vi "ReversedEngineering UpdateAttributes.vi"(1 "ClassPath/LvClassRef":variant, 2 "NewAttributes":string="Sträng:STRING\nMittCluster:CLUSTER", 3 "ClassInfo":cluster{"ClassNamn":string, "ClassPath":path}[](array[cluster]), 5 "error in (no error)":errorcluster, 6 "Don't Prompt (False)":bool, 7 "Attributes":T1[](array[typedef]), 8 "Stereotype":string) -> (18 "Cancel":bool=TRUE, 19 "error out":errorcluster)   [LabVIEW 2012] (continued)
"Recessed Up Triangle"=3618, "Reciprocal"=1059, "Reciprocal Of Pi"=2017, "Reciprocal Of e"=2021, "Rectangular Stop Button"=3128, "Refnum to Path"=1424, "Refnum to Session"=2306, "Register Event Callback"=2078, "Register For Events"=2065, "Register Session"=2319, "Release Notifier"=9102, "Release Queue"=9109, "Replace Array Subset"=3910, "Replace Substring"=3913, "Request Deallocation"=1610, "ResetSys"=1976, "Reshape Array"=2055, "Reverse 1D Array"=1900, "Reverse String"=1537, "Right Arrow"=3825, "Right Bow Valve"=21765, "Right Bow Valve 1"=3705, "Right Bow Valve 2"=3805, "Right Down Elbow"=3817, "Right Down Elbow 1"=3717, "Right Pump"=3719, "Right Pump 1"=3819, "Right Rect Valve"=3804, "Right Rect Valve 1"=3704, "Right Rect Valve 2"=21764, "Right Tee"=3715, "Right Tee 1"=3815, "Right Up Elbow"=3814, "Right Up Elbow 1"=3714, "Ring Constant"=2008, "Rocker"=21002, "Rotary Feeder"=3830, "Rotate"=1082, "Rotate 1D Array"=1906, "Rotate Left With Carry"=1606, "Rotate Right With Carry"=1607, "Rotate String"=1536, "Round Button"=3100, "Round LED"=21012, "Round LED 1"=3120, "Round Light"=3104, "Round Push Button"=3112, "Round Push Button 2"=3118, "Round Radio Button"=3106, "Round Stop Button"=3127, "Round To +Infinity"=1076, "Round To -Infinity"=1075, "Round To Nearest"=1055, "Rydberg Constant (/m)"=2031, "Scale By Power Of 2"=1074, "Scan From File"=2082, "Scan From String"=2080, "Scan String For Tokens"=8101, "Scan Value"=1534, "Search 1D Array"=1901, "Search and Replace String"=3914, "Search/Split String"=1538, "Secant"=1203, "Seconds To Date/Time"=1309, "Seek"=1409, "Select"=1516, "Send"=1977, "Send Notification"=9104, "SendCmds"=1978, "SendDataBytes"=1979, "SendIFC"=1980, "SendLLO"=1982, "SendList"=1981, "SendSetup"=1983, "Session to Refnum"=2307, "Set Menu Item Info"=9006, "Set Occurrence"=1702, "Set Variant Attribute"=8204, "Set Waveform Attribute"=8207, "SetRWLS"=1984, "SetTimeOut"=1985, "Sign"=1049, "Simple Horizontal Slide"=3003, "Simple Numeric"=2900, "Simple Numeric 1"=3029, "Simple String"=2115, "Simple Vertical Slide"=3002, "Simulation Loop"=2099, "Sinc"=1227, "Sine"=1200, "Sine & Cosine"=1220, "Single Selection Listbox"=21200, "Size Handle"=1603, "Slide Switch"=21011, "Sort 1D Array"=1120, "Speed Of Light In Vacuum (m/sec)"=2028, "Split 1D Array"=1908, "Split Button"=21020, "Split Number"=1170, "Split Signals"=2351, "Spreadsheet String To Array"=1539, "Square Button"=3101, "Square LED"=3121, "Square LED 1"=21013, "Square Light"=3105, "Square Push Button"=3113, "Square Push Button 2"=3119, "Square Radio Button"=3107, "Square Root"=1060, "Stacked Sequence Structure"=2000, "Standard ListBox"=3202, "State Diagram"=2051, "Static VI Reference"=2084, "Stop"=1350, "Stop Button"=21230, "String Constant"=2007, "String Control"=3200, "String Control 1"=21701, "String Indicator"=3201, "String Indicator 1"=21702, "String Length"=1502, "String Subset"=1503, "String To Byte Array"=1608, "String To IP"=1711, "String To Path"=1078, "String to Tag"=1830, "Strip Path"=1420, "SubPanel"=21810, "SubPanel (Classic)"=21811, "Subtract"=1051, "Swap Bytes"=1162, "Swap Vector Element"=1912, "Swap Words"=1163, "TCP Close Connection"=1713, "TCP Create Listener"=1717, "TCP Flattened Read"=1718, "TCP Flattened Write"=1719, "TCP Flex Read"=1720, "TCP Flex Write"=1721, "TCP Network Connection Refnum"=3407, "TCP Open Connection"=1715, "TCP Read"=1716, "TCP Wait On Listener"=1712, "TCP Write"=1714, "Tab Constant"=2012, "Tab Control"=3332, "Tab Control 1"=3330, "Table"=3301, "Table 1"=21202, "Table 2"=21212, "Tag Attribute Ring"=2063, "Tag Constant"=2089, "Tag Control"=21742, "Tag Control 1"=3302, "Tag Indicator"=21743, "Tag Indicator 1"=3303, "Tag to String"=1831, "Tangent"=1202, "Tank"=3020, "Tank 1"=21006, "Temporary Directory"=1435, "TestSRQ"=1986, "TestSys"=1987, "Text & Pict Ring"=21603, "Text & Pict Ring 1"=3016, "Text Button"=21015, "Text Ring"=21601, "Text Ring 1"=3014, "Thermometer"=21007, "Thermometer 1"=3021, "Thick Chiseled Line"=3630, "Thick Line"=3629, "Thick Line with Arrow"=3631, "Thick Lowered Box"=3635, "Thin Chiseled Line"=3627, "Thin Line"=3626, "Thin Line with Arrow"=3628, "Threshold 1D Array"=1909, "Tick Count (ms)"=1300, "Time Stamp Constant"=2068, "Time Stamp Control"=5555, "Time Stamp Control 1"=21913, "Time Stamp Indicator"=5556, "Time Stamp Indicator 1"=21914, "Timed Loop"=5570, "To Byte Integer"=1140, "To Double Precision Complex"=1152, "To Double Precision Float"=1147, "To Extended Precision Complex"=1154, "To Extended Precision Float"=1149, "To Long Integer"=1142, "To Lower Case"=1189, "To More Generic Class"=8017, "To More Specific Class"=8016, "To OLE Variant"=8002, "To Quad Integer"=1155, "To Single Precision Complex"=1151, "To Single Precision Float"=1146, "To Time Stamp"=5560, "To Unsigned Byte Integer"=1143, "To Unsigned Long Integer"=1145, "To Unsigned Quad Integer"=1156, "To Unsigned Word Integer"=1144, "To Upper Case"=1188, "To Variant"=8201, "To Word Integer"=1141, "Traditional DAQ Channel"=21733, "Traditional DAQ Channel 1"=3320, "Traditional DAQ Channel Constant"=2085, "Transpose 2D Array"=1902, "Tree"=21793, "Trigger"=1988, "TriggerList"=1989, "Two Button Dialog"=1341, "Type Cast"=1166, "Type and Creator"=1434, "UDP Close"=1726, "UDP Multicast Open"=1727, "UDP Network Connection Refnum"=3418, "UDP Open"=1723, "UDP Read"=1724, "UDP Write"=1725, "Unbundle"=2048, "Unbundle By Name"=2058, "Unflatten From String"=1161, "Unflatten From XML"=8401, "Uniform Dbl Waveform"=3312, "Uniform Int16 Waveform"=3313, "Unregister For Events"=2076, "Unregister Session"=2320, "Up Arrow"=3823, "Up Bow Valve"=3703, "Up Bow Valve 1"=21763, "Up Bow Valve 2"=3803, "Up Rect Valve"=21762, "Up Rect Valve 1"=3702, "Up Rect Valve 2"=3802, "Up Tee"=3812, "Up Tee 1"=3712, "User Item"=3506, "VI Library"=1425, "VI Refnum"=3422, "VISA Assert Interrupt Signal"=2309, "VISA Assert Trigger"=1929, "VISA Assert Utility Signal"=2310, "VISA Clear"=1927, "VISA Close"=1922, "VISA Disable Event"=1940, "VISA Discard Events"=1941, "VISA Enable Event"=1942, "VISA Find Resource"=1923, "VISA Flush I/O Buffer"=2302, "VISA GPIB Command"=2315, "VISA GPIB Control ATN"=2316, "VISA GPIB Control REN"=2304, "VISA GPIB Pass Control"=2317, "VISA GPIB Send IFC"=2318, "VISA In 16"=1930, "VISA In 32"=1944, "VISA In 8"=1936, "VISA Lock"=1993, "VISA Map Address"=1932, "VISA Map Trigger"=2311, "VISA Memory Allocation"=1997, "VISA Memory Free"=1998, "VISA Move"=2303, "VISA Move In 16"=1948, "VISA Move In 32"=1991, "VISA Move In 8"=1946, "VISA Move Out 16"=1949, "VISA Move Out 32"=1992, "VISA Move Out 8"=1947, "VISA Open"=2308, "VISA Out 16"=1931, "VISA Out 32"=1945, "VISA Out 8"=1937, "VISA Peek 16"=1934, "VISA Peek 32"=1995, "VISA Peek 8"=1938, "VISA Poke 16"=1935, "VISA Poke 32"=1996, "VISA Poke 8"=1939, "VISA Read"=1925, "VISA Read STB"=1928, "VISA Read To File"=2313, "VISA Refnum to Session"=2300, "VISA Resource Name"=21737, "VISA Resource Name Constant"=3421, "VISA Set I/O Buffer Size"=2301, "VISA Status Description"=1924, "VISA USB Control In"=2086, "VISA USB Control Out"=2087, "VISA Unlock"=1994, "VISA Unmap Address"=1933, "VISA Unmap Trigger"=2312, "VISA VXI Cmd or Query"=2305, "VISA Wait on Event"=1943, "VISA Write"=1926, "VISA Write From File"=2314, "VISA resource name"=3409, "Variant"=3310, "Variant To Data"=8003, "Variant To Flattened String"=8203, "Vert Line"=3822, "Vert Pipe"=3716, "Vert Pipe 1"=3816, "Vert Rocker"=21740, "Vertical Fill Slide"=21014, "Vertical Fill Slide 1"=3009, "Vertical Graduated Bar"=21107, "Vertical Pointer Slide"=21017, "Vertical Pointer Slide 1"=3007, "Vertical Progress Bar"=21104, "Vertical Slide"=3004, "Vertical Slide Switch"=21741, "Vertical Slide Switch 1"=3115, "Vertical Smooth Box"=3634, "Vertical Switch"=3109, "Vertical Toggle Switch"=21005, "Vertical Toggle Switch 1"=3111, "Volume Info"=1414, "Wait (ms)"=1302, "Wait For Activity"=1722, "Wait For Front Panel Activity"=1328, "Wait Until Next ms Multiple"=1327, "Wait for GPIB RQS"=1952, "Wait on Notification"=9105, "Wait on Notification from Multiple"=9106, "Wait on Occurrence"=1701, "WaitSRQ"=1990, "Waveform Chart"=3501, "Waveform Chart 1"=21717, "Waveform Chart 2"=21010, "Waveform Graph"=21703, "Waveform Graph 1"=3504, "While Loop"=2003, "While Loop 1"=2352, "White Space?"=1125, "Write Device"=1431, "Write File"=1408, "XY Graph"=3500, "XY Graph 1"=21716, "Xmath Script"=9022]
            n131 = Unbundle By Name(w370) -> ("BaseClassType"=w360:i16[], "OrgCtrl"=w365:refnum<vi>)
            n132 = property class="VI"(reference=w365, error in=w364) -> ("Callees' Names"=w362:string[])  [unwired: 2 out]
            n133 = Array Size(array=w362) -> (size(s)=w361:i32)
            n134 = while {
              tunnel: [w397] -> w374
              tunnel: w362 -> [w382] mode=indexing
              tunnel: [w396] -> w363
              tunnel: w361 -> [w393]
              tunnel: w360 -> [w385]
              i -> [w394]
              stop <- w392 stop-if-true
              n135 = call <resource>:"CommonVIs_UmlOpenVIRef.vi"("ViPath/ViName"=w382) -> ("error out"=w381:errorcluster, "vi reference"=w380:refnum<vi>)  [unwired: 3 in, 6 out]
              n136 = Increment(x=w394) -> (x+1=w395:i32)
              n137 = Greater Or Equal?(x=w395, y=w393) -> (x >= y?=w383:bool)
              n138 = property class="VI"(reference=w380, error in=w381) -> (reference out=w399:refnum<vi>, error out=w398:errorcluster, "VI Path"=w397:path, "Front Panel"=w391:refnum<vi>)
              n139 = property class="Pnl"(reference=w391) -> ("Controls[]"=w390:refnum<vi>[])  [unwired: 1 in, 2 out]
              n140 = Index Array(array=w390) -> (element=w389:refnum<vi>)  [unwired: 1 in]
              n141 = property class="Ctl"(reference=w389) -> ("Type Descriptor"=w388:i16[], "Label.Text"=w387:string)  [unwired: 1 in, 2 out]
              n142 = Close Reference(reference=w399, error in (no error)=w398) -> (error out=w396:errorcluster)
              n143 = call <resource>:"ReversedEngineering TypeDescNonNameDepentent.vi"("Type DescriptorNameDependent"=w388, "LabelText"=w387) -> ("Type DescriptorNonNameDependent"=w386:i16[])  [unwired: 17 out]
              n144 = Equal?(x=w385, y=w386) -> (x = y?=w384:bool)
              n145 = Or(x=w383, y=w384) -> (x .or. y?=w392:bool)
            }
            n146 = Unbundle By Name(w370) -> ("NewCluster"=w375:refnum<vi>)
            n147 = New VI Object(vi object class=w376, owner refnum=w375, style=w377, position/next to=cluster{"Horizontal":i16, "Vertical":i16} {"Horizontal"=0, "Vertical"=0}, 6:w374, 8:w363) -> (object refnum=w378:refnum<vi>, 0:w372:errorcluster)  [unwired: 2 out]
            n148 = property class="Clust"(reference=w378, error in=w372, "Label.Visible"=TRUE) -> (reference out=w368:refnum<vi>, error out=w366:errorcluster)
            n149 = Build Array(w368) -> (w367:refnum<vi>[])
            n150 = Bundle By Name(cluster=w370, "AddedCtrls"=w367) -> (w369:T4)
          }
          frame "GetOrgCtrlMembers" {
            (unwired) CommonVIs_AttributeDataType."UINT8" ("AttributeDataType")
            (unwired) CommonVIs_AttributeDataType."UINT8" ("type")
            n151 = Unbundle By Name(w408) -> ("OrgCluster"=w412:refnum<vi>)
            n152 = property class="Clust"(reference=w412, error in=w409) -> (error out=w410:errorcluster, "Controls[]"=w406:refnum<vi>[])  [unwired: 1 out]
            n153 = call <resource>:"ReversedEngineering GetClassAttrubutes.vi"("CtlRefnum"=w412, "error in (no error)"=w410) -> ("attributeInfo"=w414:T8[], "error out"=w411:errorcluster)  [unwired: 1 in, 15 out]
            n154 = Unbundle By Name(w408) -> ("AddedCtrls"=w407:refnum<vi>[], "OrgClusterMembers"=w401:T10)
            n155 = Array Size(array=w407) -> (size(s)=w403:i32)
            n156 = Index Array(array=w401) -> (element=w400:T11)  [unwired: 1 in]
            n157 = for {
              tunnel: w414 -> [w423] mode=indexing
              tunnel: [w421] -> w402 mode=indexing
              tunnel: w400 -> [w417]
              n158 = Unbundle By Name(w423) -> ("name"=w422:string, "dimension"=w419:i32, "type"=w418:T2)
              n159 = To Word Integer(number=w419) -> (16bit integer=w416:i16)
              n160 = To Lower Case(string=w422) -> (all lower case string=w420:string)
              n161 = Bundle(cluster=w417, "name"=w420, "AttributeDataType"=w418, "Dims"=w416) -> (w421:T11)
            }
            n162 = Delete From Array(array=w406, length=w403, index=0) -> (array with subset deleted=w405:refnum<vi>[])  [unwired: 1 out]
            n163 = Bundle By Name(cluster=w408, "OrgClusterCtrls"=w405, "OrgClusterMembers"=w402) -> (w413:T4)
          }
          frame "ParseNewAttribute" {
            n164 = call <vilib>:"Trim Whitespace.vi"("string"=w434) -> ("trimmed string"=w431:string)  [unwired: 1 in]
            n165 = Empty Array?(array=w424) -> (empty?=w425:bool)
            n166 = Spreadsheet String To Array(delimiter (Tab)="\n", format string="%s", spreadsheet string=w431, array type (2D Dbl)=string[] []) -> (array=w429:string[])
            n167 = case shown="False" w425 {
              tunnel: w429 -> [_ w441]
              tunnel: [w438 w440] -> w428
              tunnel: w426 -> [_ w439]
              tunnel: w424 -> [w438 _]
              frame False {
              }
              frame True {
                n168 = call <resource>:"ReversedEngineering_AttributeToDataType.vi"("ClassInfo"=w439, "Array"=w441) -> ("Attributes"=w440:T1[])
              }
            }
            n169 = Bundle By Name(cluster=w436, "Attributes"=w428) -> (w435:T4)
          }
          frame "None?" {
            n170 = Unbundle By Name(w445) -> ("AddedCtrls"=w453:refnum<vi>[], "Attributes"=w454:T1[])  [unwired: 1 out]
            n171 = Array Size(array=w453) -> (size(s)=w452:i32)
            n172 = Array Size(array=w454) -> (size(s)=w451:i32)
            n173 = Equal To 0?(x=w452) -> (x = 0?=w450:bool)
            n174 = Equal To 0?(x=w451) -> (x = 0?=w449:bool)
            n175 = Compound Arithmetic op=AND(w450, w449, invert FALSE ("value")) -> (w443:bool)
            n176 = Bundle By Name(cluster=w445, "AutoUpdate"=w443) -> (w444:T4)
            n177 = case shown="True" w443 {
              tunnel: w444 -> [w456 w460]
              tunnel: [w456 w459] -> w448
              tunnel: w446 -> [_ w457]
              frame False {
              }
              frame True {
                n178 = case shown="False" w457 {
                  frame False {
                    n179 = disable-structure shown="Disabled" {
                      frame Disabled {
                        n180 = One Button Dialog(message="Since no attributes where found,\nA dummy attribute has been created.\nA class attribute (Cluster) has to hold at least one element.") -> ()  [unwired: 2 out]
                      }
                      frame Enabled {
                      }
                    }
                  }
                  frame True {
                  }
                }
                n181 = Bundle By Name(cluster=w460, "Attributes"=T1[] [{"Name"="None", "DataType"=enum."BOOL", "ArrayDim"=0, "CtrlPath"=path "", "DataTypeString"="", "AccessScope"=enum."public", "InitialData"=variant}]) -> (w459:T4)
              }
            }
          }
          frame "AddControls" {
            n182 = Unbundle By Name(w471) -> ("WaveformControl"=w470:path)
            n183 = Unbundle By Name(w471) -> ("OrgClusterMembers"=w466:T10, "Attributes"=w479:T1[], "NewCluster"=w486:refnum<vi>, "AddedCtrls"=w482:refnum<vi>[])
            n184 = Unbundle By Name(w471) -> ("OrgCtrl"=w474:refnum<vi>, "OrgClusterCtrls"=w477:refnum<vi>[])
            n185 = Unbundle By Name(w471) -> ("NewCtrl"=w475:refnum<vi>, "NewCluster"=w473:refnum<vi>, "AddedCtrls"=w476:refnum<vi>[])  [unwired: 1 out]
            n186 = Index Array(array=w476) -> (element=w478:refnum<vi>)  [unwired: 1 in]
            n187 = for {
              tunnel: w486 -> [w515]
              shift-right: [w523] -> _
              shift-left: w478 -> [w516]
              shift-right: [w519] -> w484
              shift-left: w485 -> [w517]
              tunnel: [w523] -> w480 mode=indexing
              tunnel: w479 -> [w518] mode=indexing
              shift-left: w478 -> [w514]
              tunnel: w466 -> [w511]
              tunnel: w477 -> [w508]
              tunnel: w475 -> [w507]
              tunnel: w474 -> [w506]
              tunnel: w473 -> [w505]
              shift-right: [w504] -> _
              shift-left: i32[] [] -> [w503]
              tunnel: w470 -> [w491]
              tunnel: [w488] -> w467 mode=indexing
              i -> [w490]
              n188 = Unbundle By Name(w518) -> ("Name"=w492:string, "DataType"=w499:T2, "ArrayDim"=w501:i32, "CtrlPath"=w513:path)
              n189 = To Lower Case(string=w492) -> (all lower case string=w502:string)
              n190 = Equal?(x=w499, y=CommonVIs_AttributeDataType."TypeDef" ("AttributeDataType")) -> (x = y?=w496:bool)
              n191 = Equal?(x=w499, y=CommonVIs_AttributeDataType."LabVIEW Class" ("AttributeDataType")) -> (x = y?=w497:bool)
              n192 = Bundle(w502, "DataType"=w499, "ArrayDim"=w501) -> (w510:cluster{string, "DataType":T2, "ArrayDim":i32})  [unwired: 1 out]
              n193 = call <resource>:"ReversedEngineering FindAttributeToCopy.vi"("OrgClusterMembers"=w511, "Cluster"=w510, "AlreadyUSedControls"=w503) -> ("index of element"=w489:i32)  [unwired: 16 out]
              n194 = Equal?(x=w490, y=w489) -> (x = y?=w488:bool)
              n195 = Greater Or Equal To 0?(x=w489) -> (x >= 0?=w509:bool)
              n196 = Or(x=w496, y=w497) -> (x .or. y?=w495:bool)
              n197 = Compound Arithmetic op=AND(w509, invert w495) -> (w487:bool)
              n198 = case shown="False" w487 {
                tunnel: [w539 w732] -> w520
                tunnel: w517 -> [w538 w727]
                tunnel: w516 -> [w537 w744]
                tunnel: w515 -> [w536 _]
                tunnel: w514 -> [w534 _]
                tunnel: w499 -> [w532 _]
                tunnel: w513 -> [w531 _]
                tunnel: [w528 w708] -> w512
                tunnel: w501 -> [w527 _]
                tunnel: w508 -> [_ w746]
                tunnel: w489 -> [_ w711]
                tunnel: w507 -> [_ w723]
                tunnel: w506 -> [_ w733]
                tunnel: w505 -> [_ w721]
                tunnel: w503 -> [w529 w712]
                tunnel: [w529 w710] -> w504
                tunnel: w492 -> [w525 _]
                tunnel: w491 -> [w524 _]
                frame False {
                  (unwired) CommonVIs_AttributeDataType."UINT8" ("DataType")
                  # "Create New Control"
                  n199 = case shown="1.." w527 {
                    selector: w527 -> [_ w549]
                    tunnel: w538 -> [w545 w552]
                    tunnel: w537 -> [w544 _]
                    tunnel: w536 -> [w546 w553]
                    tunnel: [w546 w548] -> w526
                    tunnel: [w545 w551] -> w535
                    tunnel: w534 -> [_ w550]
                    tunnel: [w544 w550] -> w533
                    frame 0, Default {
                    }
                    frame 1.. {
                      w557 = refnum<vi> refnum  # Array
                      w556 = 21608 items=[".NET Refnum"=3441, "Absolute Value"=1054, "Access Rights"=1412, "ActiveX Container"=2072, "Add"=1050, "Add Array Elements"=1903, "Agitator"=3831, "AllSpoll"=1960, "And"=1061, "And Array Elements"=1911, "Append True/False String"=1511, "Application Refnum"=3412, "Array"=3300, "Array 1"=21608, "Array Constant"=2070, "Array Max & Min"=1907, "Array Size"=1809, "Array Subset"=2044, "Array To Cluster"=1168, "Array To Spreadsheet String"=1540, "Array of Strings to Path"=1422, "Atmospheric Tank"=3070, "Atmospheric Tank 1"=21751, "Automation Close"=8001, "Automation Open"=8000, "Automation Refnum"=3410, "Avogadro Constant (1/mol)"=2030, "Base 10 Logarithm Of e"=2022, "Bin"=3073, "Bin 1"=21755, "Bluetooth Close Connection"=9148, "Bluetooth Create Listener"=9151, "Bluetooth Discover"=9152, "Bluetooth Network Connection Refnum"=3468, "Bluetooth Open Connection"=9153, "Bluetooth Read"=9149, "Bluetooth Wait On Listener"=9147, "Bluetooth Write"=9150, "Boolean Array To Number"=1815, "Boolean To (0,1)"=1167, "Build Array"=2041, "Build Cluster Array"=2047, "Build Path"=1419, "Build Waveform"=2066, "Bundle"=2049, "Bundle By Name"=2057, "Byte Array To String"=1609, "Byte Stream File Refnum"=3408, "Call By Reference Node"=3901, "Call Chain"=1999, "Call Library Function Node"=2062, "Cancel Button"=3131, "Cancel Button 1"=21739, "Cancel Notification"=9107, "Carriage Return Constant"=2010, "Case Structure"=2001, "Cast Unit Bases"=1079, "Check Valve"=3833, "Checkbox"=3117, "Class Specifier Constant"=2094, "Classic Radio Buttons"=22003, "Close File"=1405, "Close Reference"=8011, "Cluster"=21607, "Cluster 1"=3400, "Cluster Constant"=2071, "Cluster To Array"=1169, "Code Interface Node"=2050, "Color Box"=3013, "Color Box Constant"=2120, "Color Box Thin Border"=2905, "Color Ramp"=3022, "Combo Box"=3304, "Combo Box 1"=21604, "Combo Box Constant"=2088, "Complex Conjugate"=1048, "Complex To Polar"=1045, "Complex To Re/Im"=1044, "Compound Arithmetic"=2200, "Compressor"=3832, "Concatenate Strings"=2040, "Conditional Disable Structure"=2064, "Constructor Node"=3904, "Control Help Window"=1353, "Control Online Help"=1355, "Control Refnum"=3419, "Convert Unit"=2059, "Conveyer"=3827, "Copy"=1416, "Cosecant"=1204, "Cosine"=1201, "Cotangent"=1205, "Create User Event"=2073, "Current VI's Menubar"=9000, "Current VI's Path"=1426, "DAQmx Analog Trigger Source"=21774, "DAQmx Analog Trigger Source 1"=21951, "DAQmx Analog Trigger Source 2"=3336, "DAQmx Analog Trigger Source Constant"=2119, "DAQmx Device Name"=21950, "DAQmx Device Name 1"=21773, "DAQmx Device Name 2"=3318, "DAQmx Device Name Constant"=2093, "DAQmx Global Channel"=21770, "DAQmx Global Channel 1"=21957, "DAQmx Global Channel 2"=3443, "DAQmx Global Channel Constant"=3430, "DAQmx Physical Channel"=21954, "DAQmx Physical Channel 1"=3335, "DAQmx Physical Channel 2"=21777, "DAQmx Physical Channel Constant"=2118, "DAQmx Scale Name"=21775, "DAQmx Scale Name 1"=3317, "DAQmx Scale Name 2"=21952, "DAQmx Scale Name Constant"=2116, "DAQmx Switch"=3337, "DAQmx Switch 1"=21776, "DAQmx Switch 2"=21953, "DAQmx Switch Constant"=2121, "DAQmx Task Name"=21778, "DAQmx Task Name 1"=21959, "DAQmx Task Name 2"=3442, "DAQmx Task Name Constant"=3434, "DAQmx Terminal"=21781, "DAQmx Terminal 1"=3319, "DAQmx Terminal 2"=21955, "DAQmx Terminal Constant"=2117, "Data Log File Refnum"=3402, "DataSocket Close"=1085, "DataSocket Open"=1084, "DataSocket Read"=1086, "DataSocket Refnum"=3417, "DataSocket Write"=1087, "Database Variant To Data"=8004, "Date/Time To Seconds"=1308, "Decimal Digit?"=1119, "Decimal String To Number"=1184, "Decimate 1D Array"=2046, "Decrement"=1058, "Default Directory"=1427, "Delete"=1417, "Delete From Array"=3912, "Delete Menu Items"=9004, "Delete Variant Attribute"=8206, "Delete Waveform Attribute"=8209, "Dequeue Element"=9113, "Destroy User Event"=2075, "DevClear"=1961, "DevClearList"=1962, "Device Control/Status"=1433, "Device Refnum"=3405, "Diagram Disable Structure"=2054, "Dial"=3050, "Dial 1"=21732, "Dialog Button"=3130, "Dialog Checkbox"=3132, "Dialog Chiseled Line"=3632, "Dialog Colored Rectangle"=3625, "Dialog Combo Box"=21917, "Dialog Horizontal Pointer Slide"=21902, "Dialog Horizontal Progress Bar"=21910, "Dialog Horizontal Slide"=21904, "Dialog Label"=21961, "Dialog Listbox"=21921, "Dialog Listbox 1"=2105, "Dialog Multicolumn Listbox"=21220, "Dialog Multiple Selection Multicolumn Listbox"=21221, "Dialog Numeric"=21919, "Dialog Path Control"=21922, "Dialog Pict Ring"=21925, "Dialog Radio Button"=3133, "Dialog Radio Buttons"=22002, "Dialog Recessed Frame"=3624, "Dialog Ring"=3060, "Dialog Spin Control"=21900, "Dialog String"=21920, "Dialog Tab Control"=3331, "Dialog Table"=21225, "Dialog Tree"=21794, "Dialog Vertical Pointer Slide"=21901, "Dialog Vertical Progress Bar"=21909, "Dialog Vertical Slide"=21903, "Digital Data"=3210, "Digital Data 1"=21216, "Digital Waveform Graph"=3511, "Digital Waveform Graph 1"=3502, "Digital Waveform Graph 2"=21718, "Divide"=1053, "Dlg CheckBox"=21924, "Dlg Horiz Scrollbar"=21905, "Dlg Numeric"=2100, "Dlg Numeric 2"=3006, "Dlg String"=2110, "Dlg Vert Scrollbar"=21906, "Down Arrow"=3824, "Down Bow Valve"=3707, "Down Bow Valve 1"=3807, "Down Bow Valve 2"=21767, "Down Rect Valve"=3706, "Down Rect Valve 1"=21766, "Down Rect Valve 2"=3806, "Down Tee"=3718, "Down Tee 1"=3818, "EOF"=1410, "Elementary Charge (C)"=2027, "Empty Path Constant"=2033, "Empty String Constant"=2013, "Empty String/Path?"=1112, "Enable Menu Tracking"=9002, "EnableLocal"=1963, "EnableRemote"=1964, "End of Line Constant"=2035, "Enqueue Element"=9111, "Enqueue Element At Opposite End"=9129, "Enum"=21605, "Enum 1"=3023, "Enum Constant"=2090, "Equal To 0?"=1113, "Equal?"=1102, "Error Ring Constant"=2039, "Event Callback Refnum"=3435, "Event Structure"=2052, "Exchanger"=3828, "Exclusive Or"=1063, "Exponential"=1211, "Exponential (Arg) -1"=1222, "Expression Node"=2201, "False Constant"=2006, "Feedback Node"=2353, "FieldPoint IO Point"=3439, "FieldPoint IO Point 1"=21784, "FieldPoint IO Point Constant"=3440, "File Dialog"=8081, "File Path Control"=21730, "File Path Control 1"=3203, "File Path Indicator"=21731, "File Path Indicator 1"=3204, "File/Directory Info"=1413, "FindLstn"=1965, "FindRQS"=1966, "First Call?"=1083, "Flat Box"=3602, "Flat Circle"=3605, "Flat Down Triangle"=3623, "Flat Frame"=3608, "Flat Left Triangle"=3620, "Flat Right Triangle"=3621, "Flat Round Button"=3102, "Flat Rounded Box"=3611, "Flat Sequence Structure"=2069, "Flat Square Button"=3103, "Flat Up Triangle"=3622, "Flatten To String"=1160, "Flatten To XML"=8400, "Flattened String To Variant"=8202, "Flush File"=1406, "Flush Queue"=9114, "For Loop"=2002, "Format Date/Time String"=8100, "Format Into File"=2083, "Format Into String"=2081, "Format Value"=1512, "Formula Node"=2004, "Fract/Exp String To Number"=1187, "Framed Color Box"=21019, "Framed Color Box 1"=3008, "Free Label"=2321, "Furnace"=3829, "GPIB Clear"=1954, "GPIB Initialization"=1957, "GPIB Misc"=1956, "GPIB Read"=1951, "GPIB Serial Poll"=1955, "GPIB Status"=1959, "GPIB Trigger"=1953, "GPIB Wait"=1958, "GPIB Write"=1950, "Gauge"=21009, "Gauge 1"=3040, "Generate Front Panel Activity"=1329, "Generate Occurrence"=1700, "Generate User Event"=2074, "Generic Refnum"=3428, "Generic Refnum By Reference Flatten"=3453, "Generic Refnum Deep Copy"=3447, "Generic Refnum Name"=21745, "Generic Refnum Tag"=3429, "Generic Refnum Tag By Reference Flatten"=3454, "Generic Refnum Tag Flatten"=21747, "Get Date/Time In Seconds"=1303, "Get Date/Time String"=1600, "Get Help Window Status"=1354, "Get Menu Item Info"=9005, "Get Menu Selection"=9001, "Get Menu Short Cut Info"=9007, "Get Notifier Status"=9103, "Get Queue Status"=9110, "Get Variant Attribute"=8205, "Get Waveform Attribute"=8208, "Get Waveform Components"=2067, "Global Variable"=2060, "Gravitational Constant (N m2/kg2)"=2029, "Greater Or Equal To 0?"=1114, "Greater Or Equal?"=1103, "Greater Than 0?"=1117, "Greater?"=1110, "Handle Peek"=1604, "Handle Poke"=1605, "Hex Digit?"=1123, "Hexadecimal String To Number"=1185, "HiQ-Script"=9021, "Hopper"=3072, "Hopper 1"=21754, "Horiz Line"=3821, "Horiz Pipe"=3710, "Horiz Pipe 1"=3810, "Horizontal Button Box"=3636, "Horizontal Fill Slide"=21100, "Horizontal Fill Slide 1"=3012, "Horizontal Graduated Bar"=21106, "Horizontal Pointer Slide"=3011, "Horizontal Pointer Slide 1"=21101, "Horizontal Progress Bar"=21102, "Horizontal Slide"=3010, "Horizontal Slide Switch"=3114, "Horizontal Smooth Box"=3633, "Horizontal Switch"=3108, "Horizontal Tank"=3071, "Horizontal Toggle Switch"=3110, "Horizontal Toggle Switch 1"=21700, "Hyperbolic Cosine"=1215, "Hyperbolic Sine"=1214, "Hyperbolic Tangent"=1216, "IMAQ Session"=3415, "IP To String"=1710, "IVI Delete Session"=8103, "IVI Logical Name"=3414, "IVI Logical Name 1"=21736, "IVI Logical Name Constant"=3420, "IVI New Session"=8102, "Implies"=1080, "In Range and Coerce"=1127, "Increment"=1057, "Index & Bundle Cluster Array"=2056, "Index Array"=2042, "Index String Array"=1531, "Initialize Array"=2053, "Insert Into Array"=3911, "Insert Menu Items"=9003, "Intensity Chart"=3509, "Intensity Chart 1"=21719, "Intensity Graph"=3510, "Intensity Graph 1"=21720, "Interleave 1D Arrays"=2045, "Interpolate 1D Array"=1905, "Inverse Cosine"=1207, "Inverse Hyperbolic Cosine"=1218, "Inverse Hyperbolic Sine"=1217, "Inverse Hyperbolic Tangent"=1219, "Inverse Sine"=1206, "Inverse Tangent"=1208, "Inverse Tangent (2 Input)"=1228, "Invoke Node"=3900, "IrDA Close Connection"=9144, "IrDA Create Listener"=9140, "IrDA Discover"=9141, "IrDA Network Connection Refnum"=3450, "IrDA Open Connection"=9142, "IrDA Read"=9145, "IrDA Wait On Listener"=9143, "IrDA Write"=9146, "Join Numbers"=1171, "Knob"=21000, "Knob 1"=3005, "LED Button"=3116, "Label"=21960, "Labeled Oblong Button"=3125, "Labeled Rectangular Button"=3124, "Labeled Round Button"=3122, "Labeled Square Button"=3123, "Left Arrow"=3826, "Left Bow Valve"=3701, "Left Bow Valve 1"=3801, "Left Bow Valve 2"=21761, "Left Down Elbow"=3811, "Left Down Elbow 1"=3711, "Left Pump"=3813, "Left Pump 1"=3713, "Left Rect Valve"=3700, "Left Rect Valve 1"=21760, "Left Rect Valve 2"=3800, "Left Tee"=3809, "Left Tee 1"=3709, "Left Up Elbow"=3708, "Left Up Elbow 1"=3808, "Less Or Equal To 0?"=1115, "Less Or Equal?"=1104, "Less Than 0?"=1118, "Less?"=1111, "Lexical Class"=1126, "Line Feed Constant"=2011, "List Directory"=1418, "Listbox"=21210, "Listbox 1"=3206, "Listbox Symbol Ring Constant"=2038, "Local Variable"=2061, "Lock Range"=1411, "Logarithm Base 10"=1210, "Logarithm Base 2"=1225, "Logarithm Base X"=1224, "Logical Shift"=1081, "Lowered Rounded Box"=3638, "MATLAB Script"=9020, "MakeAddr"=1967, "Mantissa & Exponent"=1150, "Match First String"=1532, "Match Pattern"=1535, "Match True/False String"=1533, "Max & Min"=1108, "Menu Refnum"=3413, "Menu Ring"=3018, "Menu Ring 1"=21600, "Menu-Popup Ring"=3017, "Merge Signals"=2350, "Meter"=21008, "Meter 1"=3030, "Molar Gas Constant (J/(mol K))"=2032, "Motion Resource"=3448, "Motion Resource 1"=21787, "Motion Resource Constant"=3449, "Motor"=3720, "Motor 1"=3820, "Move"=1415, "Multicolumn Listbox"=21204, "Multicolumn Listbox 1"=21205, "Multicolumn Listbox 2"=3307, "Multicolumn Listbox 3"=21214, "Multicolumn Listbox 4"=21215, "Multiple Selection Listbox"=21211, "Multiple Selection Listbox 1"=3207, "Multiple Selection Listbox 2"=3208, "Multiple Selection Listbox 3"=21201, "Multiple Selection Multicolumn Listbox"=3308, "Multiply"=1052, "Multiply Array Elements"=1904, "Natural Logarithm"=1209, "Natural Logarithm (Arg +1)"=1221, "Natural Logarithm Base"=2020, "Natural Logarithm Of 10"=2023, "Natural Logarithm Of 2"=2024, "Natural Logarithm Of Pi"=2018, "Negate"=1069, "Negative Infinity"=2019, "New Directory"=1402, "New File"=1404, "New VI"=8014, "New VI Object"=8015, "Not"=1064, "Not A Number/Path/Refnum?"=1128, "Not A Path Constant"=2034, "Not And"=1071, "Not Equal To 0?"=1116, "Not Equal?"=1105, "Not Exclusive Or"=1073, "Not Or"=1072, "Not a Refnum Constant"=2036, "Not a Tag"=2037, "Number To Boolean Array"=1814, "Number To Decimal String"=1180, "Number To Engineering String"=1183, "Number To Exponential String"=1505, "Number To Fractional String"=1506, "Number To Hexadecimal String"=1181, "Number To Octal String"=1182, "Numeric Constant"=2005, "Numeric Control"=21003, "Numeric Control 1"=3000, "Numeric Indicator"=21004, "Numeric Indicator 1"=3001, "OK Button"=21738, "OLE Variant"=3150, "Obtain Notifier"=9101, "Obtain Queue"=9108, "Occurrence Refnum"=3406, "Octal Digit?"=1129, "Octal String To Number"=1186, "Old VISA Open"=1921, "One Button Dialog"=1340, "Open Application Reference"=8012, "Open Device"=1430, "Open File"=1403, "Open File (New)"=8050, "Open Tank"=21752, "Open Tank 1"=3074, "Open VI Object Reference"=8013, "Open VI Reference"=8010, "Or"=1062, "Or Array Elements"=1910, "PPoll"=1969, "PPollConfig"=1970, "PPollUnconfig"=1971, "PassControl"=1968, "Path Constant"=2009, "Path To String"=1077, "Path Type"=1421, "Path to Array of Strings"=1423, "Pi"=2014, "Pi Divided By 2"=2016, "Pi Multiplied By 2"=2015, "Pick Line"=1510, "Pict Ring"=21602, "Pict Ring 1"=3015, "Picture"=3508, "PixMap"=3505, "PixMap (Do not touch it!!)"=3507, "Planck Constant (J/Hz)"=2026, "Platform Flat Square Button"=3134, "Plug-In Control"=21820, "Polar To Complex"=1047, "Positive Infinity"=2025, "Power Of 10"=1212, "Power Of 2"=1223, "Power Of X"=1213, "Pressure Tank"=3075, "Pressure Tank 1"=21753, "Preview Queue Element"=9112, "Printable?"=1124, "Property Node"=1920, "Pulldown Menu Ring"=3061, "Push Button"=21001, "Quit LabVIEW"=1352, "Quotient & Remainder"=1056, "Radio Buttons"=22001, "Raised Box"=3637, "Raised Box 1"=3600, "Raised Circle"=3603, "Raised Down Triangle"=3615, "Raised Frame"=3606, "Raised Left Triangle"=3612, "Raised Right Triangle"=3613, "Raised Rounded Box"=3609, "Raised Up Triangle"=3614, "Random Number (0-1)"=1070, "RcvRespMsg"=1972, "Re/Im To Complex"=1046, "Read Binary File"=8051, "Read Device"=1432, "Read File"=1407, "ReadStatus"=1973, "Receive"=1974, "ReceiveSetup"=1975, "Recessed Box"=3601, "Recessed Circle"=3604, "Recessed Down Triangle"=3619, "Recessed Frame"=3607, "Recessed Left Triangle"=3616, "Recessed Menu Ring"=3019, "Recessed Right Triangle"=3617, "Recessed Rounded Box"=3610, "Recessed Up Triangle"=3618, "Reciprocal"=1059, "Reciprocal Of Pi"=2017, "Reciprocal Of e"=2021, "Rectangular Stop Button"=3128, "Refnum to Path"=1424, "Refnum to Session"=2306, "Register Event Callback"=2078, "Register For Events"=2065, "Register Session"=2319, "Release Notifier"=9102, "Release Queue"=9109, "Replace Array Subset"=3910, "Replace Substring"=3913, "Request Deallocation"=1610, "ResetSys"=1976, "Reshape Array"=2055, "Reverse 1D Array"=1900, "Reverse String"=1537, "Right Arrow"=3825, "Right Bow Valve"=21765, "Right Bow Valve 1"=3705, "Right Bow Valve 2"=3805, "Right Down Elbow"=3817, "Right Down Elbow 1"=3717, "Right Pump"=3719, "Right Pump 1"=3819, "Right Rect Valve"=3804, "Right Rect Valve 1"=3704, "Right Rect Valve 2"=21764, "Right Tee"=3715, "Right Tee 1"=3815, "Right Up Elbow"=3814, "Right Up Elbow 1"=3714, "Ring Constant"=2008, "Rocker"=21002, "Rotary Feeder"=3830, "Rotate"=1082, "Rotate 1D Array"=1906, "Rotate Left With Carry"=1606, "Rotate Right With Carry"=1607, "Rotate String"=1536, "Round Button"=3100, "Round LED"=21012, "Round LED 1"=3120, "Round Light"=3104, "Round Push Button"=3112, "Round Push Button 2"=3118, "Round Radio Button"=3106, "Round Stop Button"=3127, "Round To +Infinity"=1076, "Round To -Infinity"=1075, "Round To Nearest"=1055, "Rydberg Constant (/m)"=2031, "Scale By Power Of 2"=1074, "Scan From File"=2082, "Scan From String"=2080, "Scan String For Tokens"=8101, "Scan Value"=1534, "Search 1D Array"=1901, "Search and Replace String"=3914, "Search/Split String"=1538, "Secant"=1203, "Seconds To Date/Time"=1309, "Seek"=1409, "Select"=1516, "Send"=1977, "Send Notification"=9104, "SendCmds"=1978, "SendDataBytes"=1979, "SendIFC"=1980, "SendLLO"=1982, "SendList"=1981, "SendSetup"=1983, "Session to Refnum"=2307, "Set Menu Item Info"=9006, "Set Occurrence"=1702, "Set Variant Attribute"=8204, "Set Waveform Attribute"=8207, "SetRWLS"=1984, "SetTimeOut"=1985, "Sign"=1049, "Simple Horizontal Slide"=3003, "Simple Numeric"=2900, "Simple Numeric 1"=3029, "Simple String"=2115, "Simple Vertical Slide"=3002, "Simulation Loop"=2099, "Sinc"=1227, "Sine"=1200, "Sine & Cosine"=1220, "Single Selection Listbox"=21200, "Size Handle"=1603, "Slide Switch"=21011, "Sort 1D Array"=1120, "Speed Of Light In Vacuum (m/sec)"=2028, "Split 1D Array"=1908, "Split Button"=21020, "Split Number"=1170, "Split Signals"=2351, "Spreadsheet String To Array"=1539, "Square Button"=3101, "Square LED"=3121, "Square LED 1"=21013, "Square Light"=3105, "Square Push Button"=3113, "Square Push Button 2"=3119, "Square Radio Button"=3107, "Square Root"=1060, "Stacked Sequence Structure"=2000, "Standard ListBox"=3202, "State Diagram"=2051, "Static VI Reference"=2084, "Stop"=1350, "Stop Button"=21230, "String Constant"=2007, "String Control"=3200, "String Control 1"=21701, "String Indicator"=3201, "String Indicator 1"=21702, "String Length"=1502, "String Subset"=1503, "String To Byte Array"=1608, "String To IP"=1711, "String To Path"=1078, "String to Tag"=1830, "Strip Path"=1420, "SubPanel"=21810, "SubPanel (Classic)"=21811, "Subtract"=1051, "Swap Bytes"=1162, "Swap Vector Element"=1912, "Swap Words"=1163, "TCP Close Connection"=1713, "TCP Create Listener"=1717, "TCP Flattened Read"=1718, "TCP Flattened Write"=1719, "TCP Flex Read"=1720, "TCP Flex Write"=1721, "TCP Network Connection Refnum"=3407, "TCP Open Connection"=1715, "TCP Read"=1716, "TCP Wait On Listener"=1712, "TCP Write"=1714, "Tab Constant"=2012, "Tab Control"=3332, "Tab Control 1"=3330, "Table"=3301, "Table 1"=21202, "Table 2"=21212, "Tag Attribute Ring"=2063, "Tag Constant"=2089, "Tag Control"=21742, "Tag Control 1"=3302, "Tag Indicator"=21743, "Tag Indicator 1"=3303, "Tag to String"=1831, "Tangent"=1202, "Tank"=3020, "Tank 1"=21006, "Temporary Directory"=1435, "TestSRQ"=1986, "TestSys"=1987, "Text & Pict Ring"=21603, "Text & Pict Ring 1"=3016, "Text Button"=21015, "Text Ring"=21601, "Text Ring 1"=3014, "Thermometer"=21007, "Thermometer 1"=3021, "Thick Chiseled Line"=3630, "Thick Line"=3629, "Thick Line with Arrow"=3631, "Thick Lowered Box"=3635, "Thin Chiseled Line"=3627, "Thin Line"=3626, "Thin Line with Arrow"=3628, "Threshold 1D Array"=1909, "Tick Count (ms)"=1300, "Time Stamp Constant"=2068, "Time Stamp Control"=5555, "Time Stamp Control 1"=21913, "Time Stamp Indicator"=5556, "Time Stamp Indicator 1"=21914, "Timed Loop"=5570, "To Byte Integer"=1140, "To Double Precision Complex"=1152, "To Double Precision Float"=1147, "To Extended Precision Complex"=1154, "To Extended Precision Float"=1149, "To Long Integer"=1142, "To Lower Case"=1189, "To More Generic Class"=8017, "To More Specific Class"=8016, "To OLE Variant"=8002, "To Quad Integer"=1155, "To Single Precision Complex"=1151, "To Single Precision Float"=1146, "To Time Stamp"=5560, "To Unsigned Byte Integer"=1143, "To Unsigned Long Integer"=1145, "To Unsigned Quad Integer"=1156, "To Unsigned Word Integer"=1144, "To Upper Case"=1188, "To Variant"=8201, "To Word Integer"=1141, "Traditional DAQ Channel"=21733, "Traditional DAQ Channel 1"=3320, "Traditional DAQ Channel Constant"=2085, "Transpose 2D Array"=1902, "Tree"=21793, "Trigger"=1988, "TriggerList"=1989, "Two Button Dialog"=1341, "Type Cast"=1166, "Type and Creator"=1434, "UDP Close"=1726, "UDP Multicast Open"=1727, "UDP Network Connection Refnum"=3418, "UDP Open"=1723, "UDP Read"=1724, "UDP Write"=1725, "Unbundle"=2048, "Unbundle By Name"=2058, "Unflatten From String"=1161, "Unflatten From XML"=8401, "Uniform Dbl Waveform"=3312, "Uniform Int16 Waveform"=3313, "Unregister For Events"=2076, "Unregister Session"=2320, "Up Arrow"=3823, "Up Bow Valve"=3703, "Up Bow Valve 1"=21763, "Up Bow Valve 2"=3803, "Up Rect Valve"=21762, "Up Rect Valve 1"=3702, "Up Rect Valve 2"=3802, "Up Tee"=3812, "Up Tee 1"=3712, "User Item"=3506, "VI Library"=1425, "VI Refnum"=3422, "VISA Assert Interrupt Signal"=2309, "VISA Assert Trigger"=1929, "VISA Assert Utility Signal"=2310, "VISA Clear"=1927, "VISA Close"=1922, "VISA Disable Event"=1940, "VISA Discard Events"=1941, "VISA Enable Event"=1942, "VISA Find Resource"=1923, "VISA Flush I/O Buffer"=2302, "VISA GPIB Command"=2315, "VISA GPIB Control ATN"=2316, "VISA GPIB Control REN"=2304, "VISA GPIB Pass Control"=2317, "VISA GPIB Send IFC"=2318, "VISA In 16"=1930, "VISA In 32"=1944, "VISA In 8"=1936, "VISA Lock"=1993, "VISA Map Address"=1932, "VISA Map Trigger"=2311, "VISA Memory Allocation"=1997, "VISA Memory Free"=1998, "VISA Move"=2303, "VISA Move In 16"=1948, "VISA Move In 32"=1991, "VISA Move In 8"=1946, "VISA Move Out 16"=1949, "VISA Move Out 32"=1992, "VISA Move Out 8"=1947, "VISA Open"=2308, "VISA Out 16"=1931, "VISA Out 32"=1945, "VISA Out 8"=1937, "VISA Peek 16"=1934, "VISA Peek 32"=1995, "VISA Peek 8"=1938, "VISA Poke 16"=1935, "VISA Poke 32"=1996, "VISA Poke 8"=1939, "VISA Read"=1925, "VISA Read STB"=1928, "VISA Read To File"=2313, "VISA Refnum to Session"=2300, "VISA Resource Name"=21737, "VISA Resource Name Constant"=3421, "VISA Set I/O Buffer Size"=2301, "VISA Status Description"=1924, "VISA USB Control In"=2086, "VISA USB Control Out"=2087, "VISA Unlock"=1994, "VISA Unmap Address"=1933, "VISA Unmap Trigger"=2312, "VISA VXI Cmd or Query"=2305, "VISA Wait on Event"=1943, "VISA Write"=1926, "VISA Write From File"=2314, "VISA resource name"=3409, "Variant"=3310, "Variant To Data"=8003, "Variant To Flattened String"=8203, "Vert Line"=3822, "Vert Pipe"=3716, "Vert Pipe 1"=3816, "Vert Rocker"=21740, "Vertical Fill Slide"=21014, "Vertical Fill Slide 1"=3009, "Vertical Graduated Bar"=21107, "Vertical Pointer Slide"=21017, "Vertical Pointer Slide 1"=3007, "Vertical Progress Bar"=21104, "Vertical Slide"=3004, "Vertical Slide Switch"=21741, "Vertical Slide Switch 1"=3115, "Vertical Smooth Box"=3634, "Vertical Switch"=3109, "Vertical Toggle Switch"=21005, "Vertical Toggle Switch 1"=3111, "Volume Info"=1414, "Wait (ms)"=1302, "Wait For Activity"=1722, "Wait For Front Panel Activity"=1328, "Wait Until Next ms Multiple"=1327, "Wait for GPIB RQS"=1952, "Wait on Notification"=9105, "Wait on Notification from Multiple"=9106, "Wait on Occurrence"=1701, "WaitSRQ"=1990, "Waveform Chart"=3501, "Waveform Chart 1"=21717, "Waveform Chart 2"=21010, "Waveform Graph"=21703, "Waveform Graph 1"=3504, "While Loop"=2003, "While Loop 1"=2352, "White Space?"=1125, "Write Device"=1431, "Write File"=1408, "XY Graph"=3500, "XY Graph 1"=21716, "Xmath Script"=9022]
                      n200 = New VI Object(vi object class=w557, owner refnum=w553, style=w556, position/next to=cluster{"Horizontal":i16, "Vertical":i16} {"Horizontal"=0, "Vertical"=0}, 4:cluster{"Width":u32, "Height":u32} {"Width"=100, "Height"=100} ("bounds"), 8:w552) -> (object refnum=w547:refnum<vi>, 0:w551:errorcluster)  [unwired: 2 out]
                      n201 = property class="Arr"(reference=w547, "Number Of Dimensions"=w549) -> (reference out=w548:refnum<vi>)  [unwired: 1 in, 1 out]
                    }
                  }
                  n202 = case shown="\"TypeDef\"" w532 {
                    selector: w532 -> [w560 _ _ _ _ _ _ _ _ _ _ _ _]
                    tunnel: w526 -> [w566 w586 w593 w603 w618 w628 w651 w655 w677 w685 w691 w698 w707]
                    tunnel: w533 -> [w565 w582 w592 w602 w617 w629 w650 w654 w676 w684 w690 w697 w706]
                    tunnel: [w563 w585 w591 w597 w608 w632 w647 w658 w673 w681 w687 w694 w703] -> w530
                    tunnel: [w561 w584 w590 w596 w607 w633 w649 w657 w675 w683 w689 w696 w705] -> w539
                    tunnel: w535 -> [w564 w583 w589 w601 w616 w627 w648 w656 w674 w682 w688 w695 w704]
                    tunnel: w531 -> [_ _ _ _ _ w624 _ w661 _ _ _ _ _]
                    tunnel: w525 -> [_ _ _ _ _ w622 _ _ _ _ _ _ _]
                    tunnel: w524 -> [_ _ _ _ _ _ _ _ _ w680 _ _ _]
                    tunnel: [_ _ _ _ w606 _ _ _ _ _ _ _ _] -> _
                    frame "UINT8".."CXT" {
                      w567 = refnum<vi> refnum  # Numeric
